vi "IQ Recorder Measurement Init.vi"(8 "error in (no error)":errorcluster, 9 "Instance (1)":i32=1 format="%.0g", 11 "VISA resource name":refnum<visa-resource-name>) -> (0 "error out":errorcluster, 3 "VISA resource name out":refnum<visa-resource-name>)   [LabVIEW 2015, in "Rohde&Schwarz CMXP GPRF.lvlib"]
doc: "Starts or restarts the measurement; the R&S CMW 500 enters the \"RUN\" state.\n\nAttribute:\nRSCMXPGPRF_ATTR_IQ_RECORDER_MEASUREMENT_INIT\n\nRemote-control command:\nINITiate:GPRF:MEAS<i>:IQRecorder"
uses:
  <instrlib>/Rohde&Schwarz CMXP GPRF/Rohde&Schwarz CMXP GPRF.lvlib
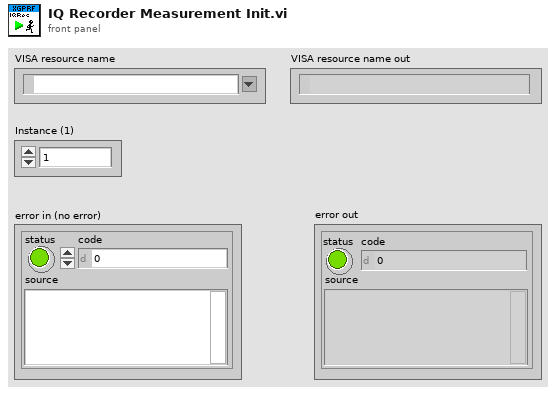
[diagram p1: front panel]
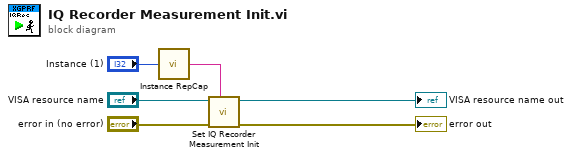
[diagram p0: block diagram]
diagram:
  n1 = call <instrlib>:"Instance RepCap.vi"("instance  in"="Instance (1)") -> ("instance out"=w1:string)
  n2 = call "Set IQ Recorder Measurement Init"("Repeated Capabilities"=w1, "error in (no error)"="error in (no error)", "instrument handle"="VISA resource name") -> ("error out"=→"error out":errorcluster, "instrument handle out"=→"VISA resource name out":refnum<visa-resource-name>)  [unwired: 7 in]
